vi "Prober_LoadUnload.vi"(8 "error in (no error)":errorcluster, 11 "VeloxTeslaProbestation in":refnum<class "VeloxTeslaProbestation.lvclass">) -> (0 "error out":errorcluster, 2 "Home or Load?":enum16{"Home", "Load"}(ring), 3 "VeloxTeslaProbestation out":refnum<class "VeloxTeslaProbestation.lvclass">)   [LabVIEW 2018, in "VeloxTeslaProbestation.lvclass"]
uses:
  VeloxTeslaProbestation.lvclass
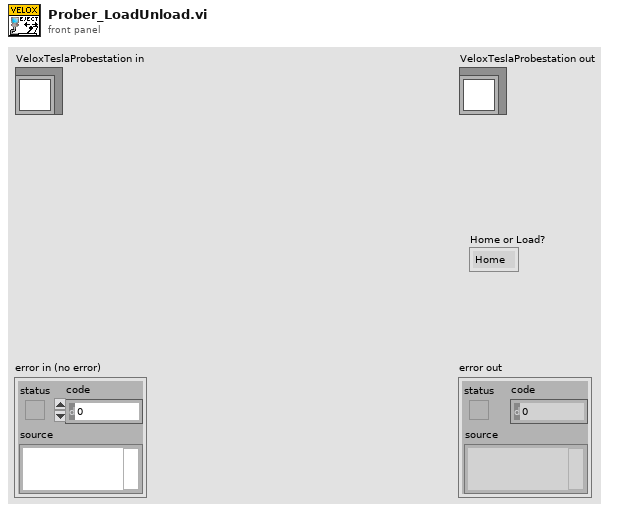
[diagram p1: front panel]
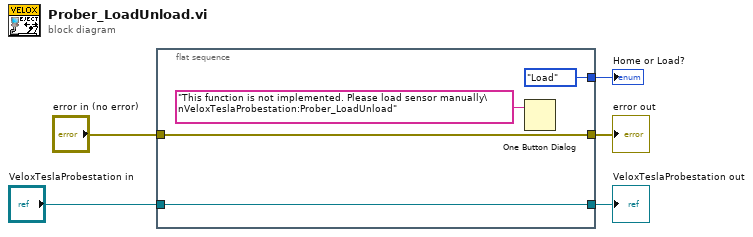
[diagram p0: block diagram]
diagram:
  n1 = flat-sequence {
    tunnel: "error in (no error)" -> [w8]
    tunnel: [w8] -> w4
    tunnel: [enum16{"Home", "Load"}."Load" ("Home or Load?")] -> w3
    tunnel: [w6] -> w2
    tunnel: "VeloxTeslaProbestation in" -> [w6]
    frame #0 {
      n2 = One Button Dialog(message="This function is not implemented. Please load sensor manually\nVeloxTeslaProbestation:Prober_LoadUnload") -> ()  [unwired: 1 in, 1 out]
    }
  }
  "error out" <- w4
  "Home or Load?" <- w3
  "VeloxTeslaProbestation out" <- w2
